vi "priv_WriteByRef.vi"(8 "error in (no error)":errorcluster, 10 "Databox_sealed":refnum<class "Databox_sealed.lvclass">, 11 "AR_Elmt":T1) -> (0 "error out":errorcluster, 1 "Write Index":bool, 2 "Data To Disp out":variant)   [LabVIEW 2020, in "UI_Actor.lvlib" / "UI_Actor.lvclass"]
uses:
  UI_Actor.lvclass
  ctl_AR_Elmt.ctl
  support/Databox.lvlibp/Databox_sealed/Databox_sealed.lvclass
  D:/Projets/STEP AT/UI Actor/support/Databox.lvlibp/Databox/Databox.lvclass
  ctl_ErrorSelector.ctl
  support/Databox.lvlibp/Databox/Read Builder name.vi
  support/Databox.lvlibp/Databox/Databox.lvclass
  support/Databox.lvlibp/TypesTools/Data/Data.lvclass
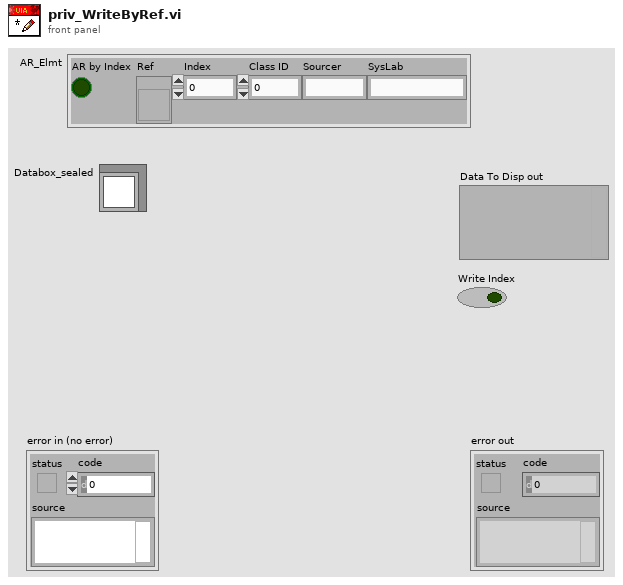
[diagram p1: front panel]
types:
  T1 = typedef "UI_Actor.lvlib/UI_Actor.lvclass/ctl_AR_Elmt.ctl" = cluster{"AR by Index":bool, "Ref":refnum<vi>, "Index":i32, "Class ID":u32, "Sourcer":string, "SysLab":string}
  T2 = typedef "ctl_ErrorSelector.ctl" = enum16{"Unknown nested UIA", "Unsupported type"}
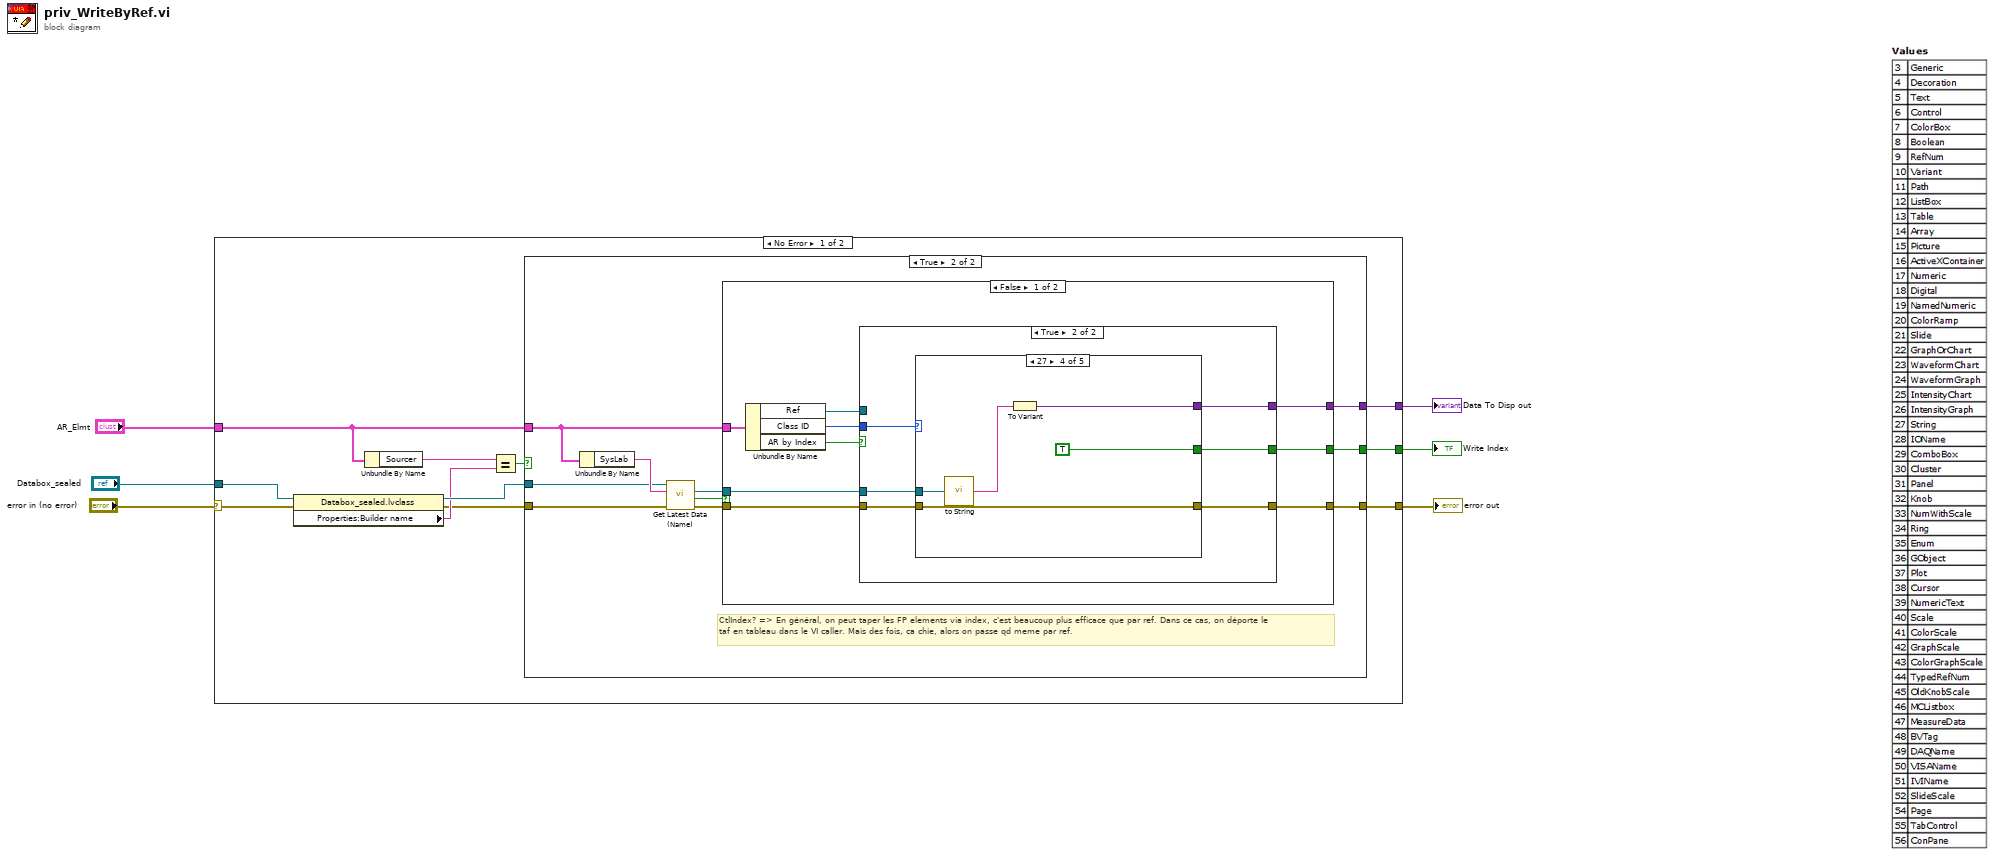
[diagram p0: block diagram]
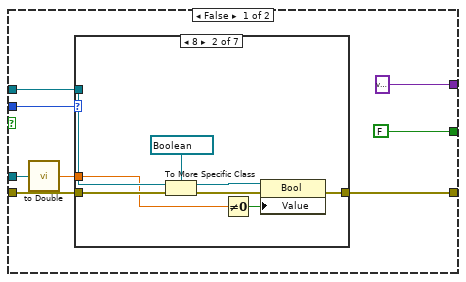
[diagram p3: hidden frame]
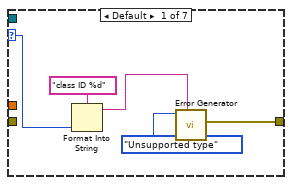
[diagram p4: hidden frame]
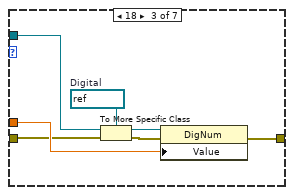
[diagram p5: hidden frame]
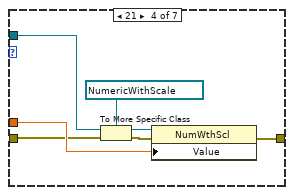
[diagram p6: hidden frame]
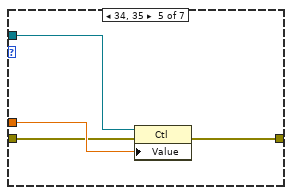
[diagram p7: hidden frame]
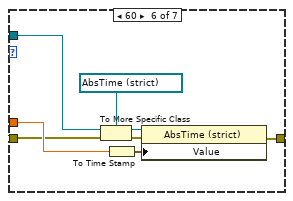
[diagram p8: hidden frame]
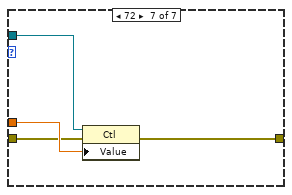
[diagram p9: hidden frame]
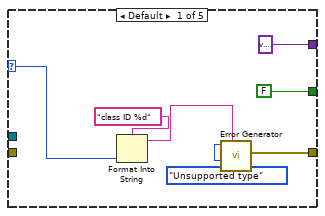
[diagram p10: hidden frame]
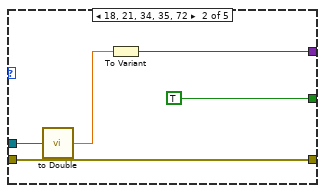
[diagram p11: hidden frame]
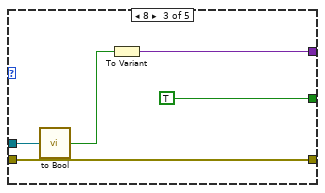
[diagram p12: hidden frame]
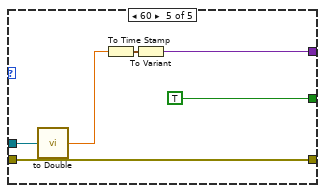
[diagram p13: hidden frame]
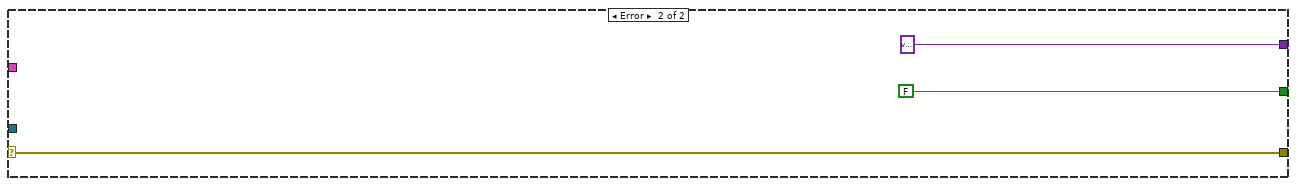
[diagram p15: hidden frame]
diagram:
  n1 = case shown="No Error" "error in (no error)" {
    selector: "error in (no error)" -> [w12 w126]
    tunnel: [w17 w126] -> w5
    tunnel: [w16 variant ("Variant")] -> w3
    tunnel: [w15 FALSE] -> w4
    tunnel: "Databox_sealed" -> [w14 _]
    tunnel: "AR_Elmt" -> [w11 _]
    frame No Error {
      n2 = property class="Databox_sealed.lvclass"(reference=w14, error in=w12) -> (reference out=w13:refnum<class "Databox_sealed.lvclass">, error out=w7:errorcluster, "Properties:Builder name"=w9:string)
      n3 = Unbundle By Name(w11) -> ("Sourcer"=w10:string)
      n4 = Equal?(x=w10, y=w9) -> (x = y?=w8:bool)
      n5 = case shown="True" w8 {
        tunnel: [w18 w28] -> w17
        tunnel: [_ w27] -> w16
        tunnel: [_ w26] -> w15
        tunnel: w13 -> [_ w21]
        tunnel: w11 -> [_ w20]
        tunnel: w7 -> [w18 w19]
        frame False {
        }
        frame True {
          # "CtlIndex? => En général, on peut taper les FP elements via index, c'est beaucoup plus efficace que par ref. Dans ce cas, on déporte le taf en tableau dans le VI caller. Mais des fois, ca chie, alors on passe qd meme par ref."
          n6 = Unbundle By Name(w20) -> ("SysLab"=w25:string)
          n7 = call "Get Latest Data (Name).vi"("error in (no error)"=w19, "Node Name"=w25, "Databox in"=w21) -> ("error out"=w24:errorcluster, "Data empty!"=w23:bool, "Latest Data"=w22:refnum<class "Data.lvclass">)  [unwired: 5 in, 1 out]
          n8 = case shown="False" w23 {
            tunnel: [w37 w123] -> w28
            tunnel: [w36 _] -> w27
            tunnel: [w35 _] -> w26
            tunnel: w20 -> [w31 _]
            tunnel: w24 -> [w30 w123]
            tunnel: w22 -> [w29 _]
            frame False {
              n9 = Unbundle By Name(w31) -> ("Ref"=w34:refnum<vi>, "Class ID"=w33:u32, "AR by Index"=w32:bool)
              n10 = case shown="True" w32 {
                tunnel: [w45 w93] -> w37
                tunnel: w33 -> [w44 w92]
                tunnel: w34 -> [w43 _]
                tunnel: w30 -> [w42 w94]
                tunnel: [variant ("Variant") w91] -> w36
                tunnel: [FALSE w90] -> w35
                tunnel: w29 -> [w39 w89]
                frame False {
                  n11 = call "to Double.vi"("Data"=w39) -> ("Double"=w38:dbl)
                  n12 = case shown="8" w44 {
                    selector: w44 -> [w50 _ _ _ _ _ _]
                    tunnel: w38 -> [_ w52 w64 w71 w76 w84 w88]
                    tunnel: [w47 w54 w62 w69 w75 w83 w87] -> w45
                    tunnel: w42 -> [_ w55 w61 w68 w73 w80 w85]
                    tunnel: w43 -> [_ w53 w60 w67 w74 w82 w86]
                    frame Default {
                      n13 = Format Into String(format string="class ID %d", w50) -> (resulting string=w46:string)  [unwired: 2 in, 1 out]
                      n14 = call "Error Generator.vi"("Details"=w46, "Error selector"=ctl_ErrorSelector."Unsupported type") -> ("error out"=w47:errorcluster)  [unwired: 9 in]
                    }
                    frame 8 {
                      n15 = To More Specific Class(target class=refnum<vi> refnum ("num 21"), reference=w53, error in=w55) -> (specific class reference=w58:refnum<vi>, error out=w57:errorcluster)
                      n16 = Not Equal To 0?(x=w52) -> (x != 0?=w51:bool)
                      n17 = property class="Bool"(reference=w58, error in=w57, "Value"=w51) -> (error out=w54:errorcluster)  [unwired: 1 out]
                    }
                    frame 18 {
                      w59 = refnum<vi> refnum  # Digital
                      n18 = To More Specific Class(target class=w59, reference=w60, error in=w61) -> (specific class reference=w65:refnum<vi>, error out=w63:errorcluster)
                      n19 = property class="DigNum"(reference=w65, error in=w63, "Value"=w64) -> (error out=w62:errorcluster)  [unwired: 1 out]
                    }
                    frame 21 {
                      n20 = To More Specific Class(target class=refnum<vi> refnum ("num 21"), reference=w67, error in=w68) -> (specific class reference=w72:refnum<vi>, error out=w70:errorcluster)
                      n21 = property class="NumWthScl"(reference=w72, error in=w70, "Value"=w71) -> (error out=w69:errorcluster)  [unwired: 1 out]
                    }
                    frame 34, 35 {
                      n22 = property class="Ctl"(reference=w74, error in=w73, "Value"=w76) -> (error out=w75:errorcluster)  [unwired: 1 out]
                    }
                    frame 60 {
                      n23 = To More Specific Class(target class=refnum<vi> refnum ("Time Stamp"), reference=w82, error in=w80) -> (specific class reference=w81:refnum<vi>, error out=w79:errorcluster)
                      n24 = To Time Stamp(1:w84) -> (0:w77:timestamp)
                      n25 = property class="AbsTime (strict)"(reference=w81, error in=w79, "Value"=w77) -> (error out=w83:errorcluster)  [unwired: 1 out]
                    }
                    frame 72 {
                      n26 = property class="Ctl"(reference=w86, error in=w85, "Value"=w88) -> (error out=w87:errorcluster)  [unwired: 1 out]
                    }
                  }
                }
                frame True {
                  n27 = case shown="27" w92 {
                    selector: w92 -> [w95 _ _ _ _]
                    tunnel: [w96 w104 w109 w114 w119] -> w93
                    tunnel: w94 -> [_ w104 w109 w114 w119]
                    tunnel: [variant ("Variant") w105 w111 w116 w121] -> w91
                    tunnel: [FALSE TRUE TRUE TRUE TRUE] -> w90
                    tunnel: w89 -> [_ w103 w108 w113 w118]
                    frame Default {
                      n28 = Format Into String(format string="class ID %d", w95) -> (resulting string=w99:string)  [unwired: 2 in, 1 out]
                      n29 = call "Error Generator.vi"("Details"=w99, "Error selector"=ctl_ErrorSelector."Unsupported type") -> ("error out"=w96:errorcluster)  [unwired: 9 in]
                    }
                    frame 18, 21, 34, 35, 72 {
                      n30 = call "to Double.vi"("Data"=w103) -> ("Double"=w102:dbl)
                      n31 = To Variant(anything=w102) -> (Variant=w105:variant)
                    }
                    frame 8 {
                      n32 = call "to Bool.vi"("Data"=w108) -> ("Boolean"=w107:bool)
                      n33 = To Variant(anything=w107) -> (Variant=w111:variant)
                    }
                    frame 27 {
                      n34 = call "to String.vi"("Data"=w113) -> ("String"=w112:string)
                      n35 = To Variant(anything=w112) -> (Variant=w116:variant)
                    }
                    frame 60 {
                      n36 = call "to Double.vi"("Data"=w118) -> ("Double"=w117:dbl)
                      n37 = To Time Stamp(1:w117) -> (0:w122:timestamp)
                      n38 = To Variant(anything=w122) -> (Variant=w121:variant)
                    }
                  }
                }
              }
            }
            frame True {
            }
          }
        }
      }
    }
    frame Error {
    }
  }
  "error out" <- w5
  "Data To Disp out" <- w3
  "Write Index" <- w4
